vi "BB_Vertical_Analysis.vi"(3 "Scored Particle Info":T1(array[cluster]), 6 "Camera Type":enum16{"206", "1011"}(ring), 9 "X Resolution":i32, 10 "Y Resolution":i32) -> ()   [LabVIEW 2012]
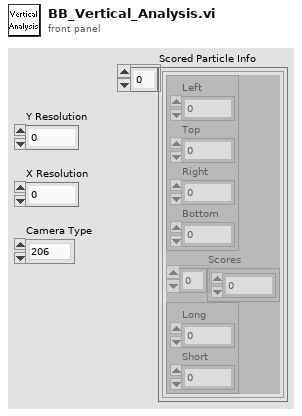
[diagram p1: front panel]
types:
  T1 = cluster{cluster{"Left":dbl, "Top":dbl, "Right":dbl, "Bottom":dbl}, "Scores":dbl[], cluster{"Long":dbl, "Short":dbl}}[]
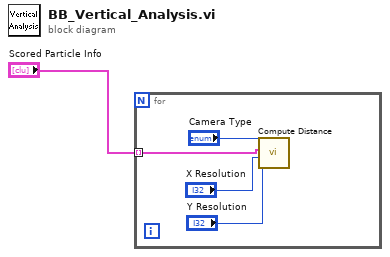
[diagram p0: block diagram]
diagram:
  n1 = for {
    tunnel: "Scored Particle Info" -> [w2] mode=indexing
    n2 = call "Compute Distance.vi"("Y Image Resolution"="Y Resolution", "X Image Resolution"="X Resolution", "Particle Scores"=w2, "Camera Type"="Camera Type") -> ()  [unwired: 5 in, 3 out]
  }
